vi "Read U32.vi"(8 "error in (no error)":errorcluster, 11 "Local Bus in":refnum<class "Local Bus.lvclass">) -> (0 "error out":errorcluster, 2 "U32":refnum<data-value>, 3 "Local Bus out":refnum<class "Local Bus.lvclass">)   [LabVIEW 2021]
uses:
  Local Bus.lvclass
  Local Bus.lvclass/Local Bus.ctl
  C:/Users/Tim/Documents/GitHub/Omni-Bus/Source/Bus_Access/Bus_Access.lvclass
  C:/Program Files (x86)/National Instruments/LabVIEW 2021/vi.lib/TSA/Abstract Data Classes/Abs_Types/Type/Abs_Type.lvclass
  C:/Users/Tim/Documents/GitHub/Omni-Bus/Source/Local Bus/Local Bus.lvclass
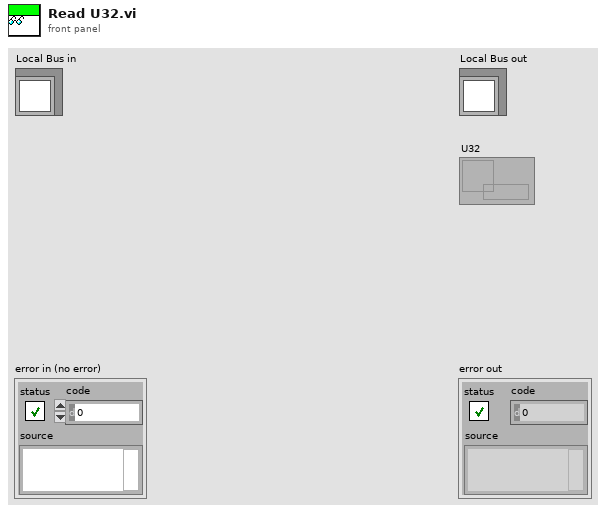
[diagram p1: front panel]
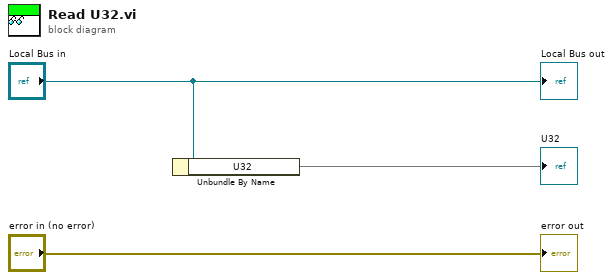
[diagram p0: block diagram]
diagram:
  n1 = Unbundle By Name("Local Bus in") -> ("U32"=→"U32")
  "error out" <- "error in (no error)"
  "Local Bus out" <- "Local Bus in"
